vi "RdID.vi"(11 "element in":T1) -> (1 "id":u32)   [LabVIEW 2019, in "MessengerM.lvlib"]
uses:
  <resource>/Channels/MessengerM/MessengerM.lvlib
  <resource>/Channels/MessengerM/Element.ctl
  <vilib>/ChannelSupport/Channel Message/Channel Message.lvclass
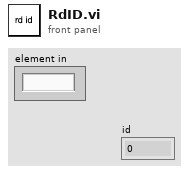
[diagram p1: front panel]
types:
  T1 = typedef "MessengerM.lvlib/Element.ctl" = string
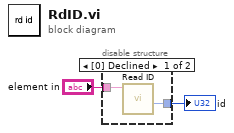
[diagram p0: block diagram]
diagram:
  n1 = disable-structure shown="[0] Declined" {
    disable-tunnel: "element in" -> [w4 _]
    disable-tunnel: [w3 _] -> w2
    frame Disabled {
      n2 = call <vilib>:"Read ID.vi"("Channel Message in"=w4) -> ("id"=w3:u32)  [unwired: 10 in]
    }
    frame Enabled {
    }
  }
  "id" <- w2
